vi "Graphs.vi"() -> ()   [LabVIEW 2018]
panel:
  out "HIGH PRESS PSIG 2":dbl(graph)
  out "Igniter (60)":dbl
  out "Thermometer":dbl(slide)=45.3739 scale=0.0..250.0
  out "HIGH PRESS PSIG":dbl
  out "HIGH PRESS PSIG":dbl(graph)
  out "LOX":dbl
  out "FUEL":dbl
  out "Chamber PSIG":dbl
  out "MV FUEL":dbl
  out "MV LOX":dbl
  out "Chamber PSIG":dbl(graph)
  out "MV Fuel/LOX PSIG":cluster{"Numeric":dbl, "Numeric":dbl}(graph)
  out "Fuel/LOX PSIG":cluster{"Numeric":dbl, "Numeric":dbl}(graph)
  out "Thrust Force lbf":dbl
  in  "stop":bool
  out "Thrust Force":dbl(graph)
  # "CSULB Vehicle Health"
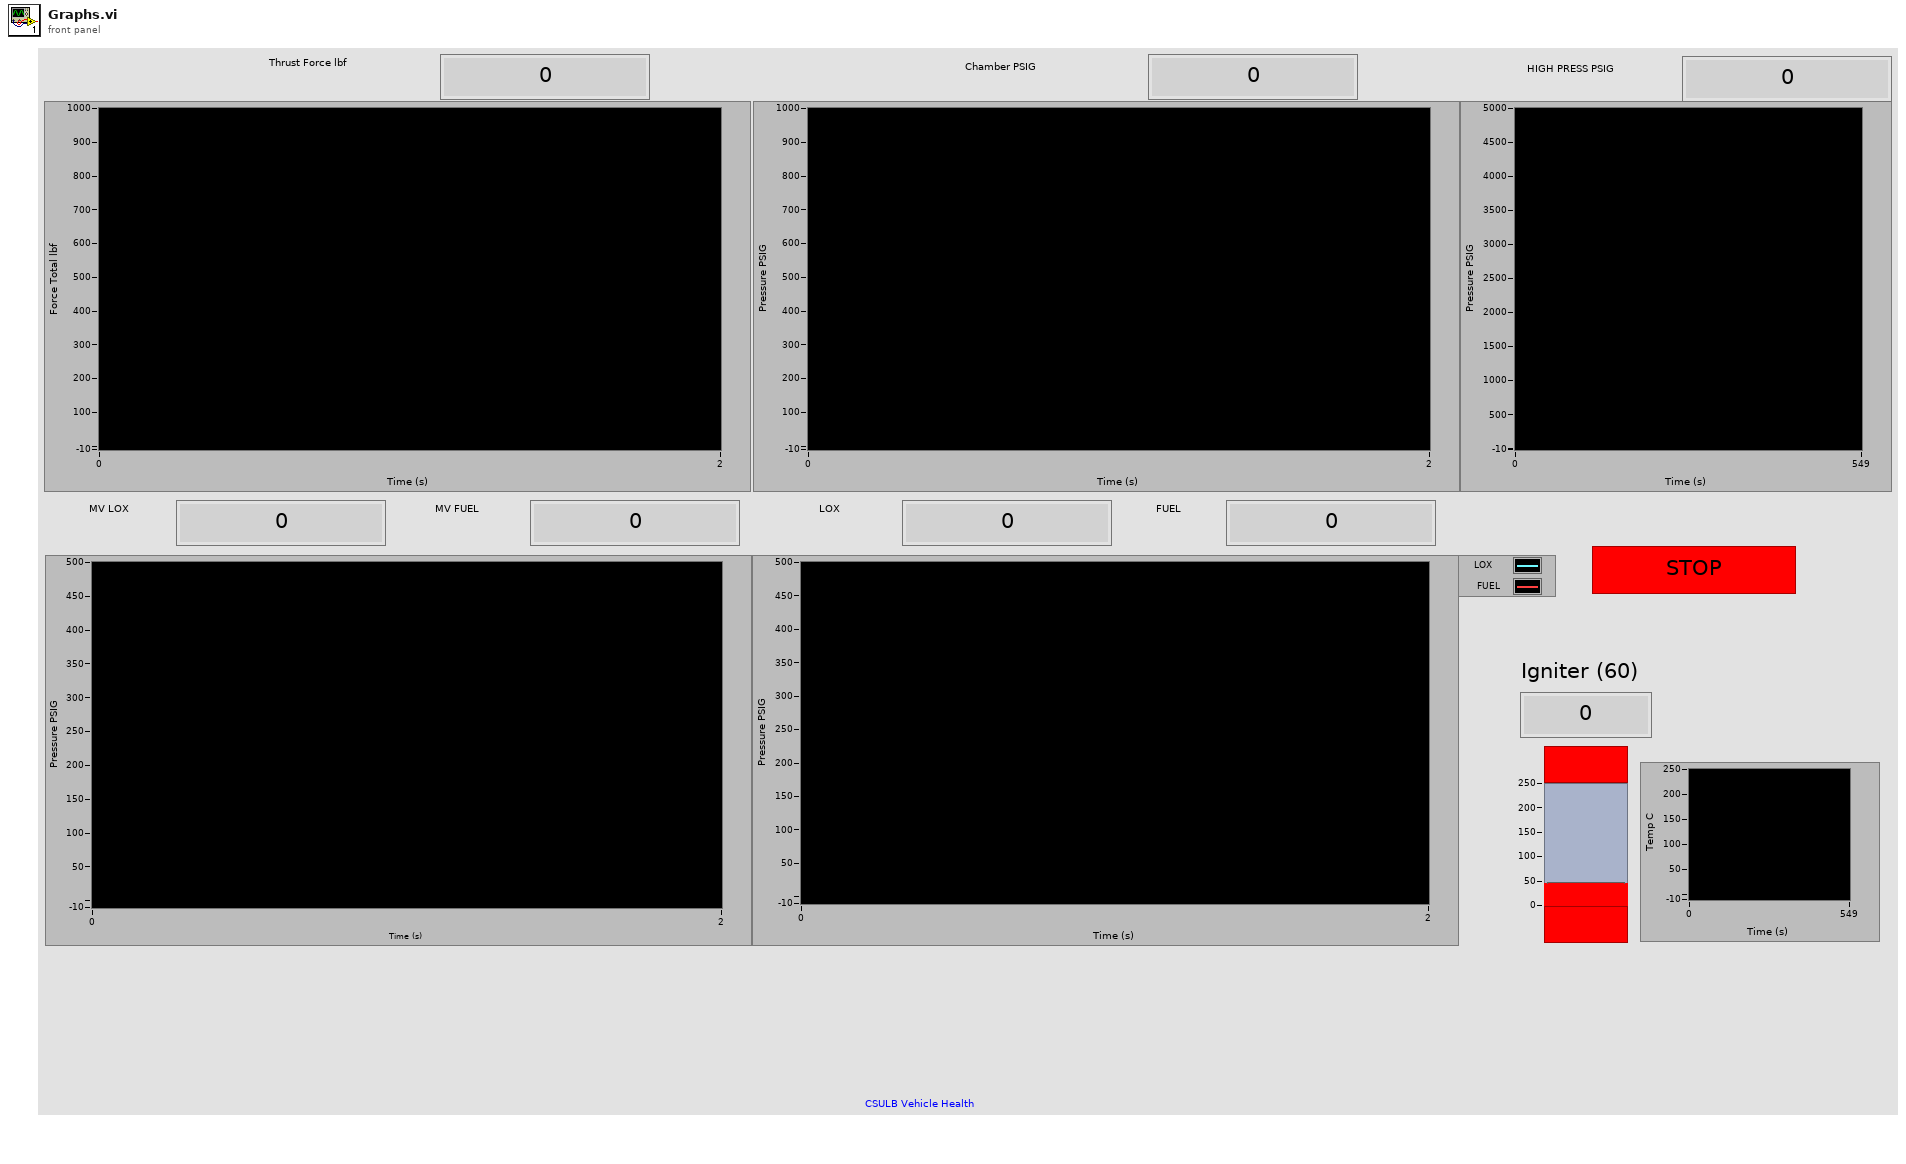
[diagram p1: front panel]
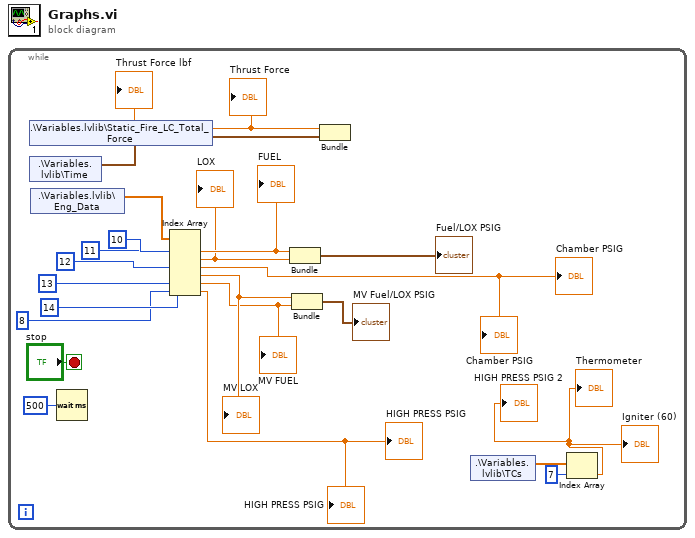
[diagram p0: block diagram]
diagram:
  n1 = while {
    stop <- "stop" stop-if-true
    n2 = shared-variable ".\\Variables.lvlib\\Static_Fire_LC_Total_Force"() -> (w19:dbl)  [unwired: 1 in, 1 out]
    "Thrust Force" <- w19
    "Thrust Force lbf" <- w19
    n3 = shared-variable ".\\Variables.lvlib\\Time"() -> (w20:timestamp)  [unwired: 1 in, 1 out]
    n4 = shared-variable ".\\Variables.lvlib\\Eng_Data"() -> (w18:dbl[])  [unwired: 1 in, 1 out]
    n5 = Wait (ms)(milliseconds to wait=u32 500) -> ()  [unwired: 1 out]
    n6 = Index Array(array=w18, index #1=10 ("index"), index #2=11 ("index"), index #3=12 ("index"), index #4=13 ("index"), index #5=14 ("index"), index #6=8 ("index")) -> (element #1=w13:dbl, element #2=w12:dbl, element #3=→"Chamber PSIG" →"Chamber PSIG":dbl, element #4=w9:dbl, element #5=w8:dbl, element #6=→"HIGH PRESS PSIG" →"HIGH PRESS PSIG":dbl)
    "MV LOX" <- w9
    "MV FUEL" <- w8
    "FUEL" <- w13
    "LOX" <- w12
    n7 = Bundle("Numeric"=w13, "Numeric"=w12) -> (→"Fuel/LOX PSIG":cluster{"Numeric":dbl, "Numeric":dbl})  [unwired: 1 in]
    n8 = Bundle("Numeric"=w9, "Numeric"=w8) -> (→"MV Fuel/LOX PSIG":cluster{"Numeric":dbl, "Numeric":dbl})  [unwired: 1 in]
    n9 = Bundle("Double"=w19, "Timestamp"=w20) -> ()  [unwired: 1 in, 1 out]
    n10 = shared-variable ".\\Variables.lvlib\\TCs"() -> (w3:dbl[])  [unwired: 1 in, 1 out]
    n11 = Index Array(array=w3, index=7) -> (element=→"Thermometer" →"Igniter (60)" →"HIGH PRESS PSIG 2":dbl)
  }
